vi "PXI-5441_Init.vi"(8 "Error In":errorcluster, 10 "Resource Name":refnum<k15>, 11 "Object in":refnum<class "PXI-5441.lvclass">) -> (0 "Error Out":errorcluster, 3 "object out":refnum<class "PXI-5441.lvclass">)   [LabVIEW 2023, in "HAL.lvlib" / "PXI-5441.lvlib" / "PXI-5441.lvclass"]
uses:
  PXI-5441.lvclass
  PXI-5441.lvclass/PXI-5441.ctl
  states/Disconnected_class/Disconnected.lvclass
  Hardware_class/Hardware.lvclass
  D:/git/HAL/Hardware_class/Hardware.lvclass
  D:/git/HAL/IFGEN_interface/IFGEN.lvclass
  D:/git/HAL/IFGEN_interface/IStates_interface/IStates.lvclass
  D:/git/HAL/PXI-5441_class/PXI-5441.lvclass
  D:/git/HAL/PXI-5441_class/IConfigurable_interface/IConfigurable.lvclass
  D:/git/HAL/PXI-5441_class/states/Disconnected_class/Disconnected.lvclass
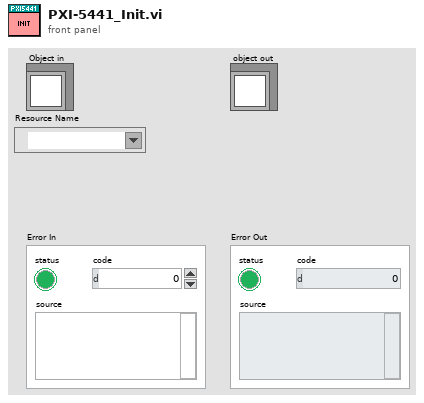
[diagram p1: front panel]
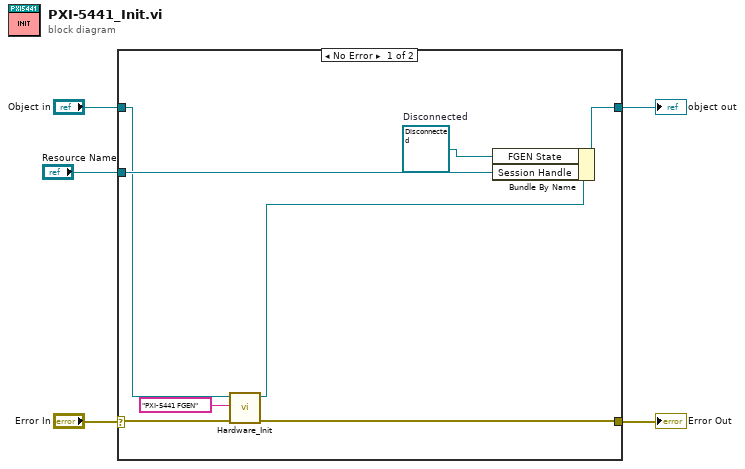
[diagram p0: block diagram]
diagram:
  n1 = case shown="No Error" "Error In" {
    selector: "Error In" -> [w13 w14]
    tunnel: [w12 w15] -> w5
    tunnel: "Object in" -> [w8 w15]
    tunnel: [w11 w14] -> w2
    tunnel: "Resource Name" -> [w10 _]
    frame No Error {
      w9 = refnum<class "Disconnected.lvclass"> refnum  # Disconnected
      n2 = call "Hardware_Init.vi"("Error In"=w13, "HW Device Name"="PXI-5441 FGEN", "object in"=w8) -> ("Error Out"=w11:errorcluster, "object out"=w6:refnum<class "PXI-5441.lvclass">)  [unwired: 7 in]
      n3 = Bundle By Name(cluster=w6, "FGEN State"=w9, "Session Handle"=w10) -> (w12:refnum<class "PXI-5441.lvclass">)
    }
    frame Error {
    }
  }
  "object out" <- w5
  "Error Out" <- w2
